vi "New.vi"(6 "rect in":T1, 7 "picture in":picture, 10 "color in":u32(colorbox)) -> (3 "Rectangle out":refnum<class "Rectangle.lvclass">, 5 "picture out":picture)   [LabVIEW 2024, in "Rectangle.lvclass"]
doc: "MIT Licence\nCopyright (c) 2024 David Grollier"
uses:
  Rectangle.lvclass
  Rectangle.lvclass/Rectangle.ctl
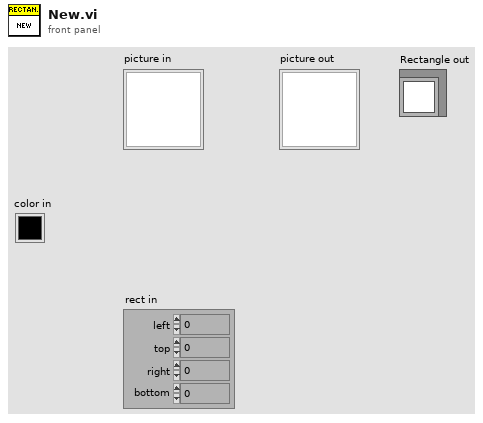
[diagram p1: front panel]
types:
  T1 = cluster{"left":i16, "top":i16, "right":i16, "bottom":i16}
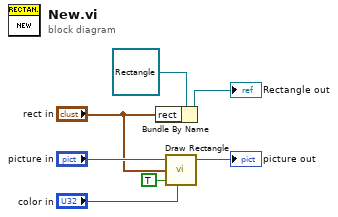
[diagram p0: block diagram]
diagram:
  n1 = Bundle By Name(cluster=refnum<class "Rectangle.lvclass"> refnum ("Rectangle in"), "rect"="rect in") -> (→"Rectangle out":refnum<class "Rectangle.lvclass">)
  n2 = call <vilib>:"Draw Rectangle.vi"("picture"="picture in", "rect"="rect in", "fill?(F)"=TRUE, "color(black)"="color in") -> ("new picture"=→"picture out":picture)  [unwired: 5 in]
